vi "信号光谱4-拟合.vi"() -> ()   [LabVIEW 2015]
uses:
  <vilib>/Utility/file.llb/Write Delimited Spreadsheet (DBL).vi
  <vilib>/Analysis/NI_AALBase.lvlib
panel:
  out "范围内？":bool[](array[boolean])
  out "w":dbl
  out "xc":dbl
  out "拟合参数":dbl[](array[numeric])
  out "best fit":dbl[](graph) caption="最佳拟合"
  out "最终存储路径":path
  in  "停止程序":bool
  in  "上升下降沿/s":dbl format="%.2p"
  in  "延时/s":dbl format="%.2p"
  in  "占空比/%":dbl=3.0 format="%.2p"
  in  "高电平/V":dbl=4.0 format="%.2p"
  in  "频率/Hz":dbl=100.0 format="%.3p"
  in  "低电平/V":dbl min=0.0 max=5.0 format="%.2p"
  out "configure error out":errorcluster
  in  "设置参数":bool
  out "output control error  4":errorcluster
  in  "低电平持续输出":bool
  in  "Output 1":bool
  out "output control error  5":errorcluster
  in  "脉冲作用时间/s":dbl=1.0
  in  "测量高电平/V":dbl=4.0
  out "output control error  2":errorcluster
  in  "测量次数":i32=1
  in  "开始测量":bool
  in  "上升下降沿":i32(ring)=1 items=["上升沿", "下降沿"]
  in  "channel输出口":i32(ring) items=["Channel 1", "Channel 2"]
  in  "输出信号波形":u16(ring) items=["Pulse"]
  out "output control error  3":errorcluster
  out "Output":bool
  in  "VISA 信号发生器":refnum<visa-resource-name>="USB0::0x1AB1::0x0641::DG4E192200870::INSTR"
  out "Spectrum":cluster{"Y":dbl[], "Y":dbl[]}[](graph)
  in  "计数器":dbl=720.0
  out "波长范围":dbl[](array[numeric])
  in  "选项卡控件":enum32{"IHR 550", "CCD"}(tab)
  in  "Move To\nTarget Positions":bool
  out "Current UniqueID":string="Mono4"
  in  "Mono ID":string(combo)="Mono1"
  in  "Connect":bool
  out "Initialized JY":bool=TRUE
  in  "Force\nInitialization":bool
  in  "Target Grating":string(combo)="2"
  out "Current Description":string="1" caption="Description"
  out "Grating Index":i32=1
  out "Current Grating":dbl=1200.0
  out "Units":string="nm"
  out "Current WL":dbl=897.9988
  out "Exit Mirror\nPosition":i32(ring)=2 items=["EntranceMirror", "ExitMirror", "Front", "Side"]
  out "Entrance Mirror\nPosition":i32(ring)=2 items=["EntranceMirror", "ExitMirror", "Front", "Side"]
  out "Units 2":string="mm"
  out "Front Entrance":dbl
  in  "Target WL":dbl=2670.0
  in  "Exit Mirror":u16(ring)=3 caption="Target Position Exit Mirror" items=["Front"=2, "Side"=3]
  in  "Entrance Mirror":u16(ring)=2 caption="Target Position\nEntrance Mirror" items=["Front"=2, "Side"=3]
  in  "Target\nFront Entrance":dbl=1.0
  in  "Commande tab":T1(tab)
  in  "Area Number to Display":i32
  in  "Reformat":bool
  in  "GAIN":u16(ring)=2 caption="Device Name" items=["High Light", "Best Dynamic Range", "High Sensitivity"]
  in  "ADC":u16(ring) caption="Device Name" items=["20 kHz       ", " 1 MHz       ", " 1 MHz Ultra "]
  in  "Number of Areas :":u16=1 min=1 step=1
  in  "Integration time (ms) :":i16=5000
  out "Uniques ID":u16(ring) items=["CCD1", "CCD2"]
  in  "Device Name":u16(ring) items=["Synapse CCD (Lateral)", "Synapse_IGA (Axial)"]
  in  "Signal type :":enum16{"TTL Rising Edge", "TTL Falling Edge"}(ring)=enum."TTL Falling Edge"
  in  "Trigger Type :":u16(ring) items=["On Start"=1, "Per Acquisition"=2]
  in  "trigSigTypeString":string
  in  "trigEventString":string
  in  "Enable InputTriggers :":bool
  in  "Number of Cleans":i32=1
  in  "MultiAcqShutterMode":i32(ring)=3 items=["Open For All Spectra"=1, "Open for Each Spectrum"=3]
  in  "Accumulations:":u16=10 min=1 step=1
  in  "Multi Accumulation mode:":bool
  out "Y Pixels:":i32=256
  out "DataSize":i32=1024
  out "X Pixels:":i32=1024
  out "Firmware\nVersion":string="V1.20 CCD_4000"
  out "initialized ?":bool=TRUE
  in  "Continuous":bool
  in  "CCD Busy":bool
  out "indicator":string="Ready !"
  in  "initialize":bool
  in  "ShutterOpen":bool=TRUE caption="Shutter enable"
  in  "Acquire":bool
  in  "Temperature":bool
  in  "Setup":bool
  in  "起始波长":dbl=2406.79
  in  "终止波长":dbl=2919.91
  out "Acq Time(ms)":u32=3401
  in  "Save Backlight":bool
  in  "cut backlight":bool
  out "backlight":bool=TRUE
  in  "Close":bool=TRUE
  out "JYCCDLib.IJYCCDReqd":refnum<k7>
  out "areas :":i32[][](array[numeric])=[[1], [1], [1], [1024], [256], [1], [256]]
  in  "Constante de condition\n(Voir l'aide contextuelle)":bool
  out "temp graph":dbl(graph)=-134.538067
  out "ADC Number":i32[](array[numeric])=[0, 1, 2, 3, 4]
  out "Gain Number":i32[](array[numeric])=[10, 11, 12, 13, 8, 2]
  out "trigAddress":i32
  out "Data":i32[][](graph)
  out "error out":errorcluster
  out "Gratings":dbl[](array[numeric])=[1200.0, 300.0]
  out "Backlight":i32[][](graph)
  out "data 2":i32[][](graph)
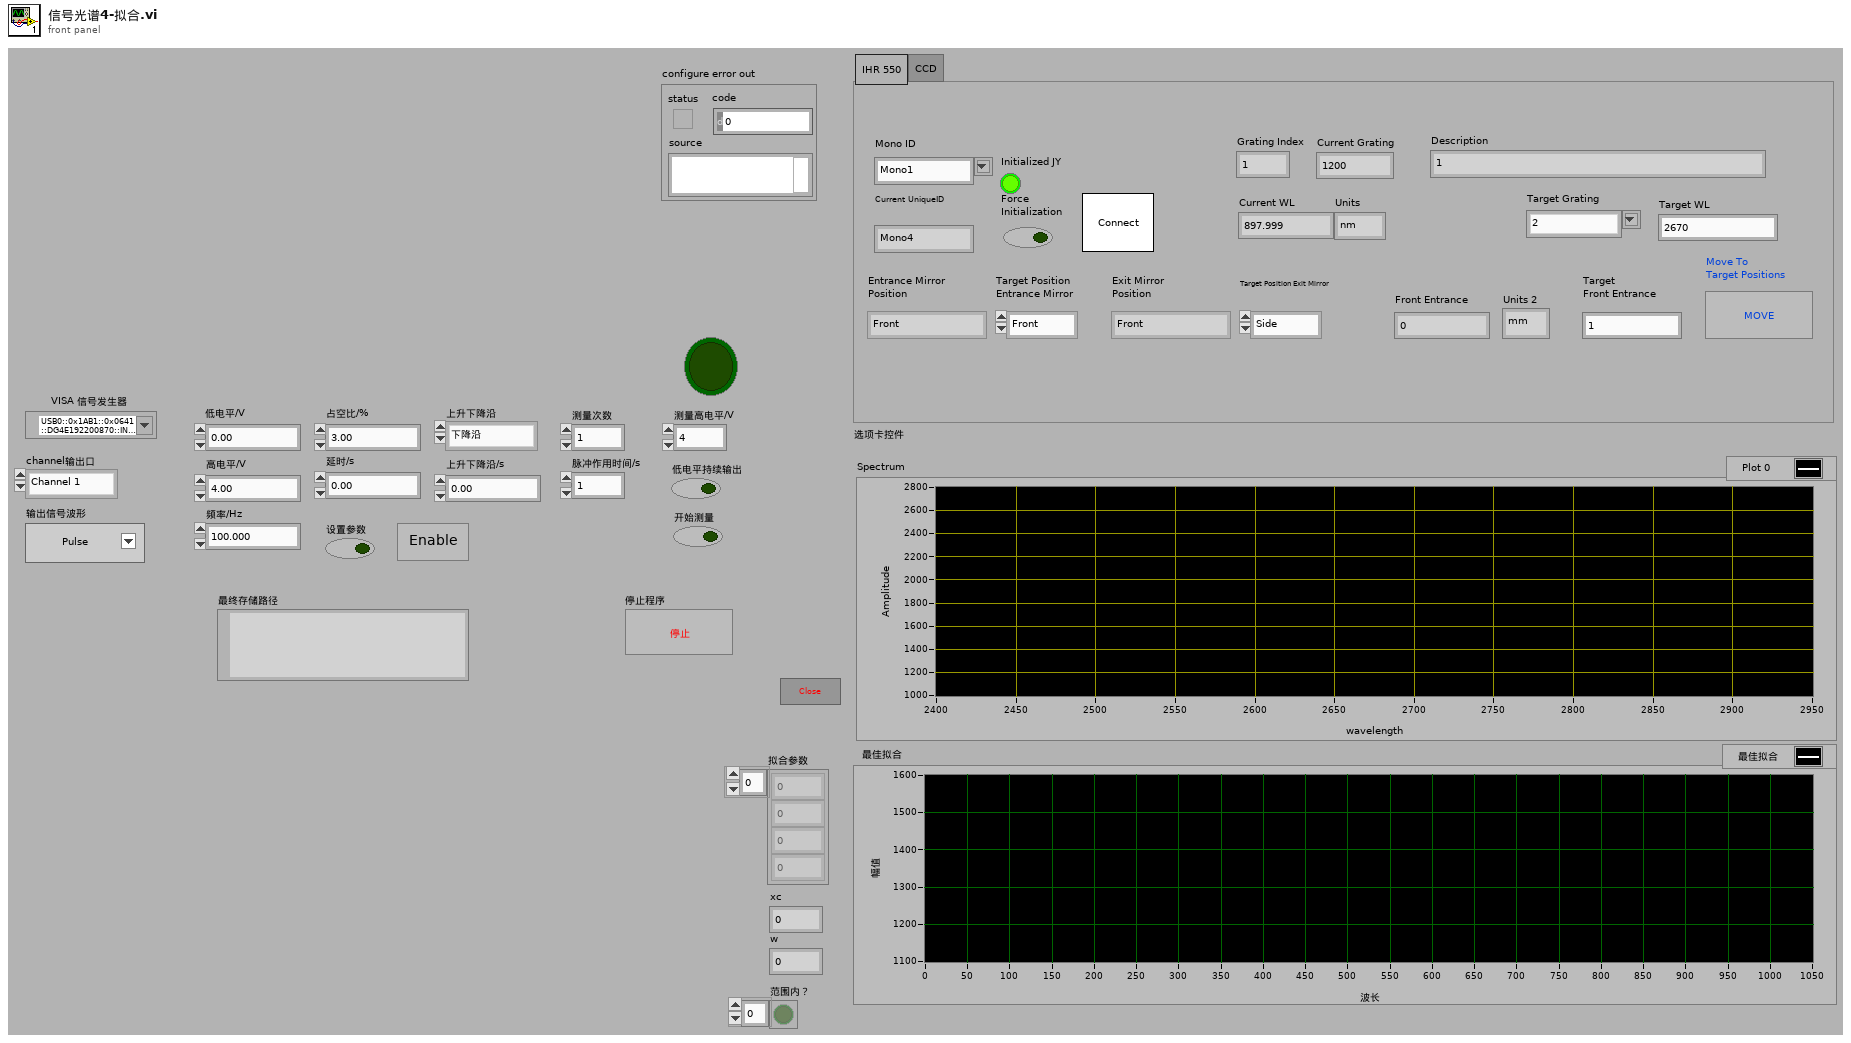
[diagram p1: front panel]
types:
  T1 = enum32{"Settings", "Trigger In", "Multi-Accu.", "Infos"}
  T2 = enum8{"Enabled", "Disabled", "Disabled and Grayed Out"}
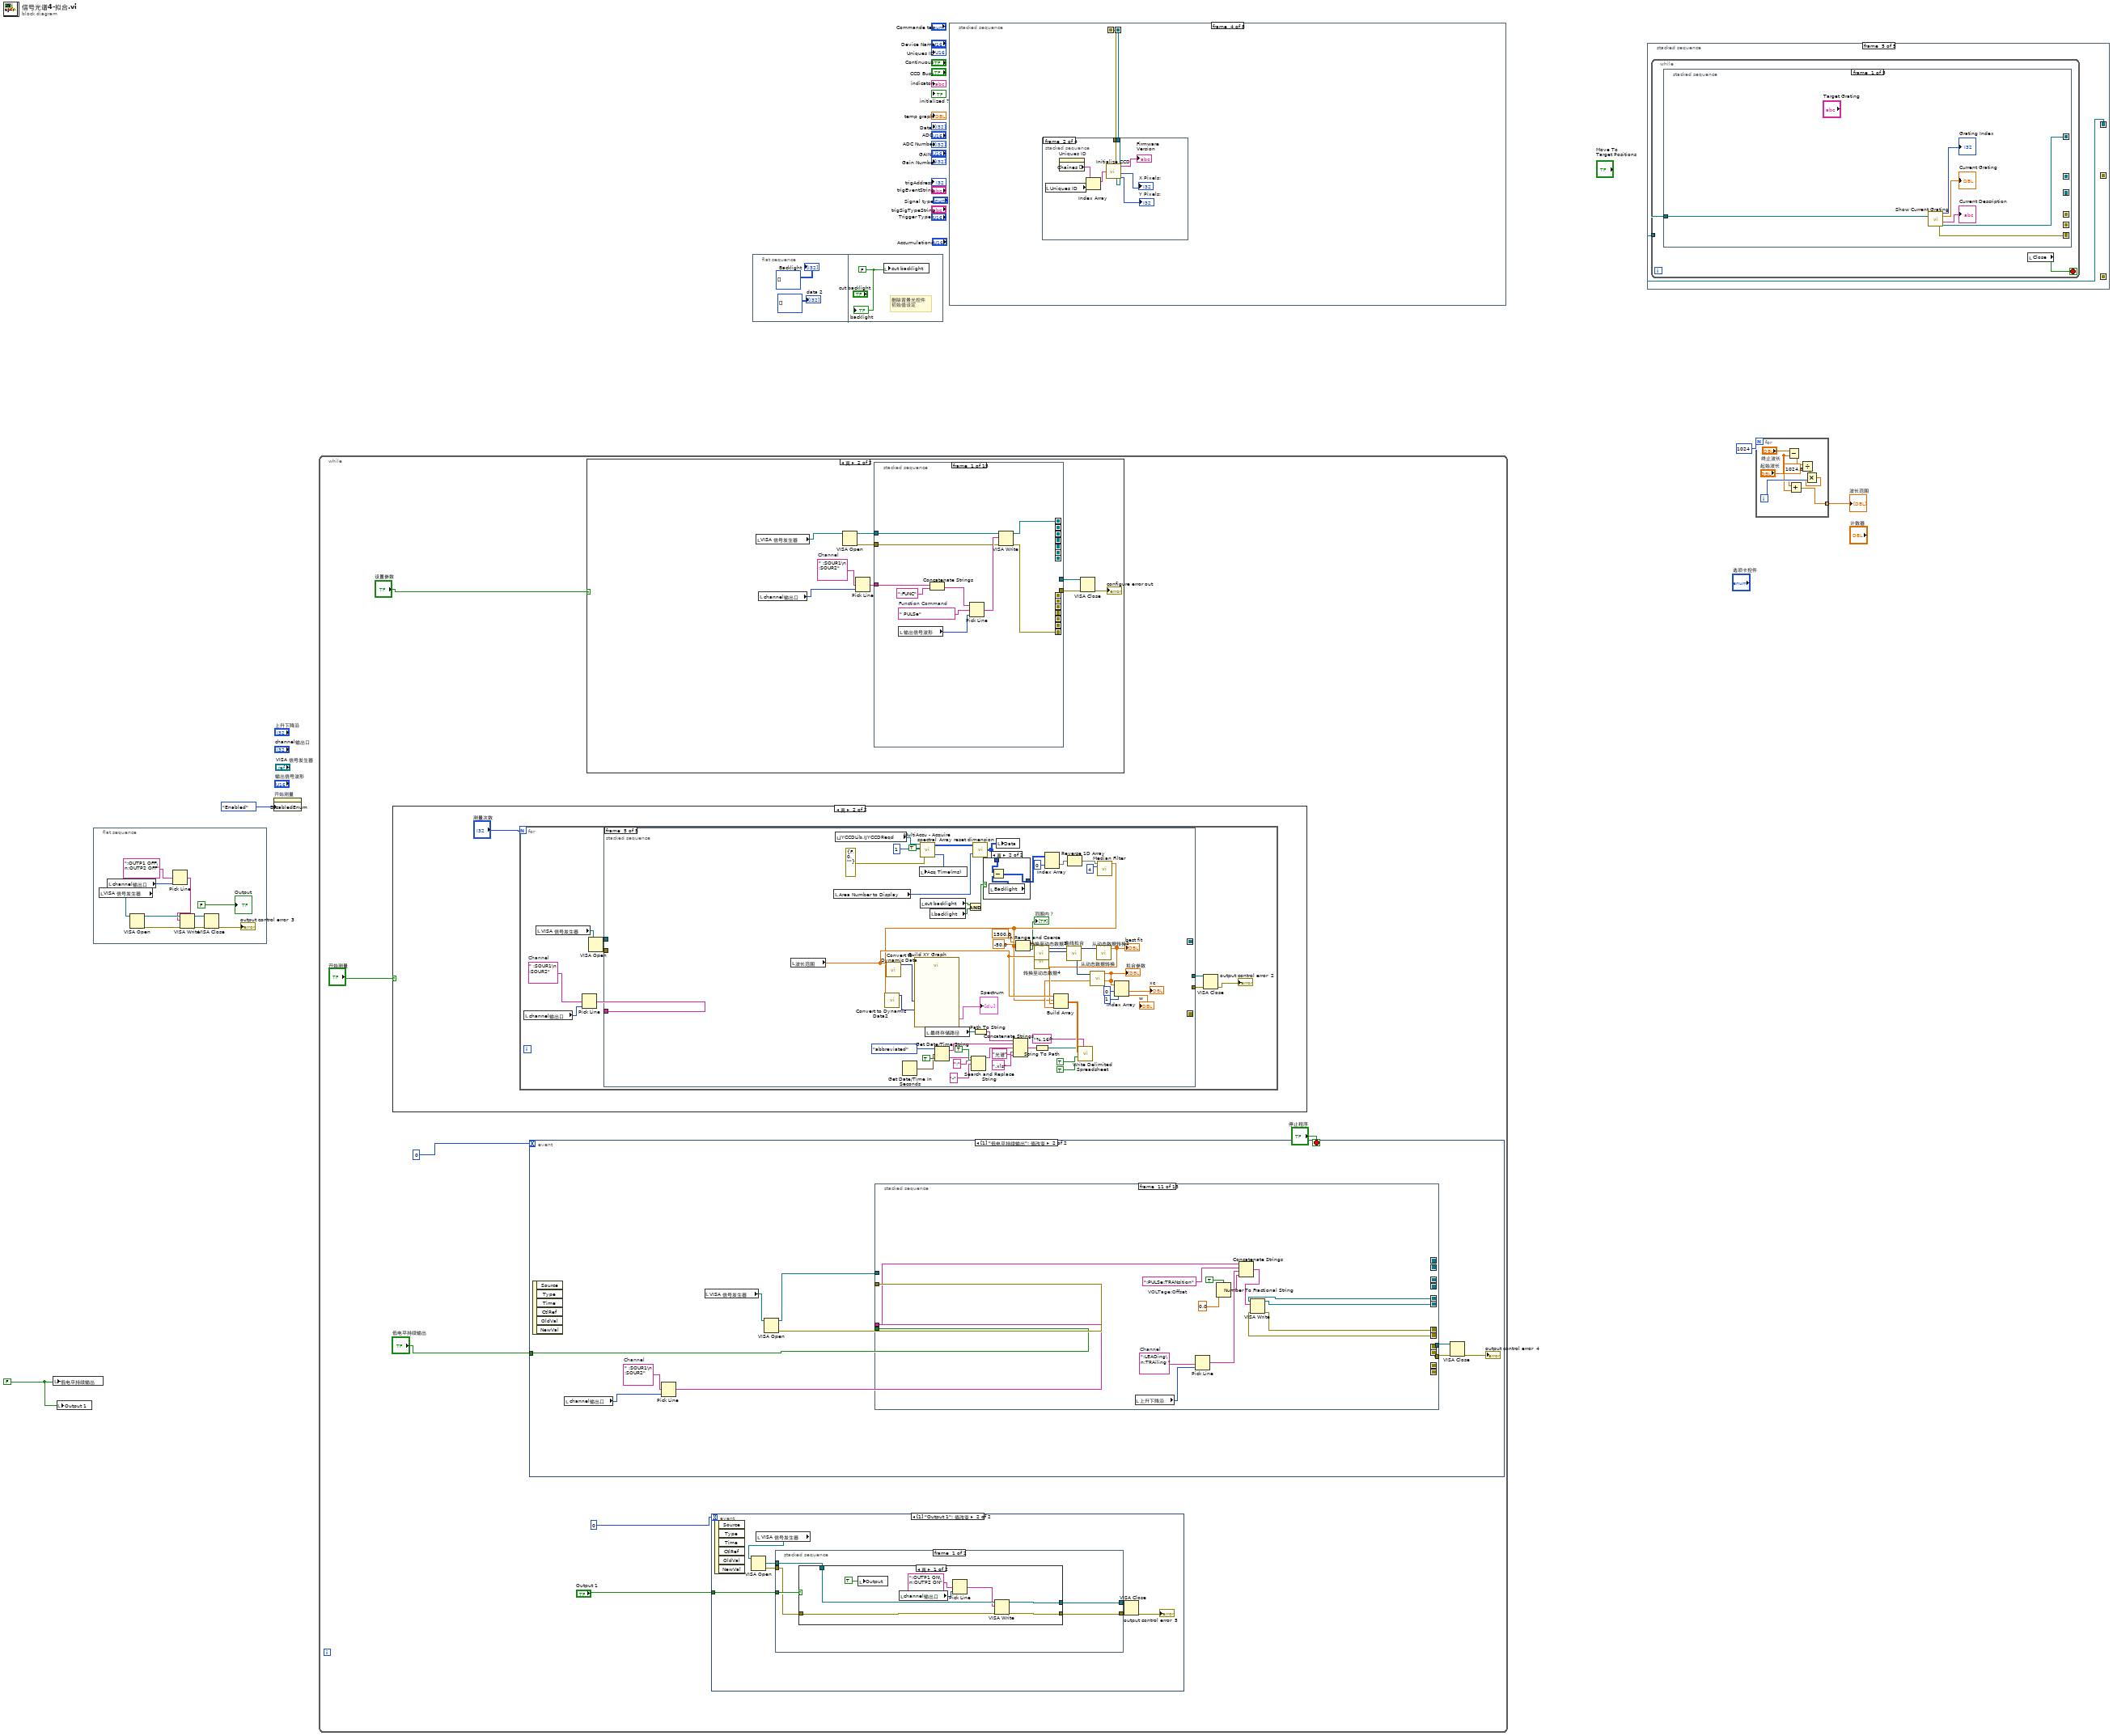
[diagram p0: block diagram]
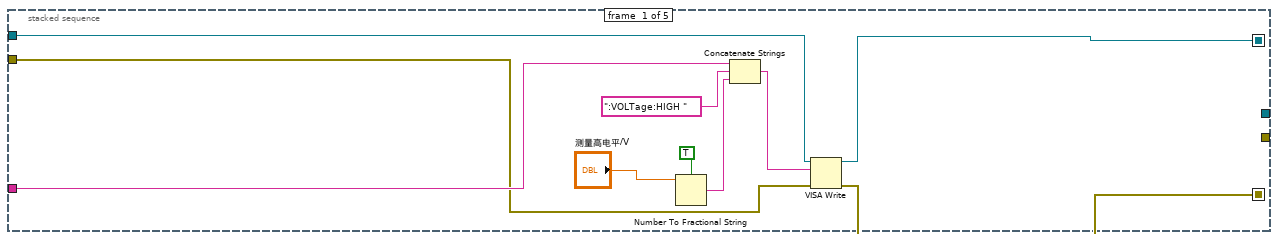
[diagram p3: hidden frame]
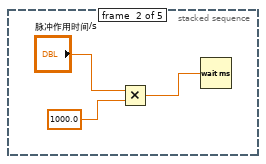
[diagram p4: hidden frame]
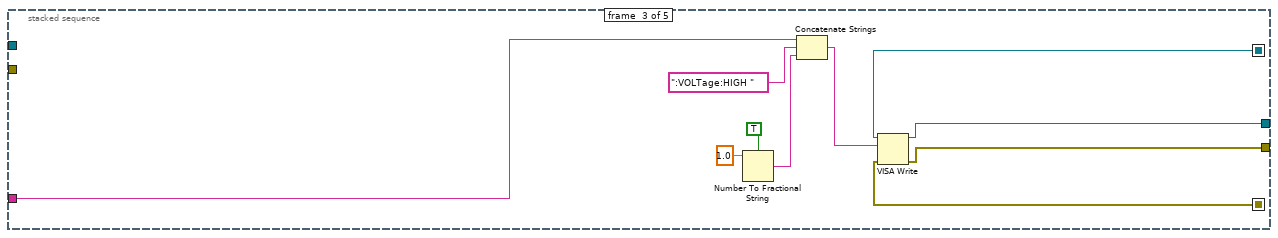
[diagram p5: hidden frame]
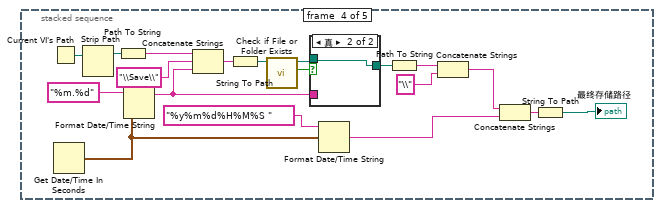
[diagram p6: hidden frame]
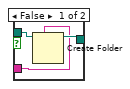
[diagram p7: hidden frame]
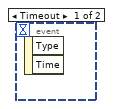
[diagram p9: hidden frame]
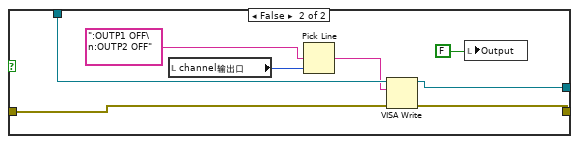
[diagram p10: hidden frame]
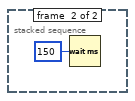
[diagram p11: hidden frame]
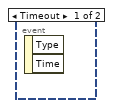
[diagram p12: hidden frame]
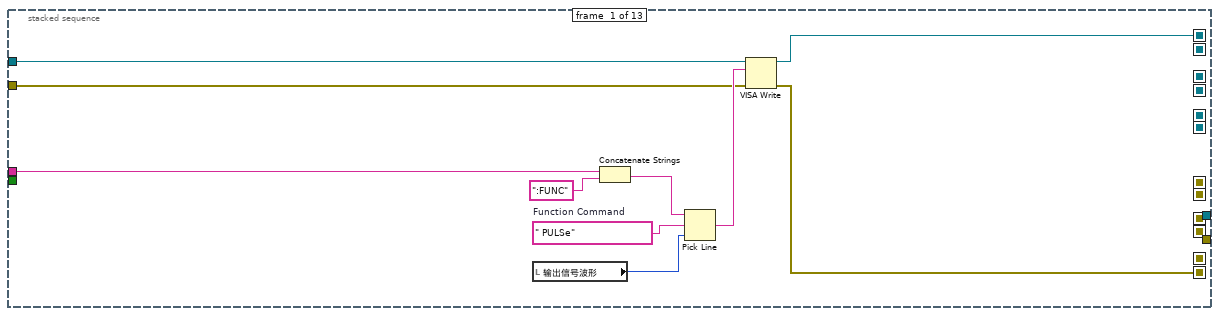
[diagram p13: hidden frame]
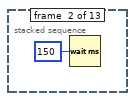
[diagram p14: hidden frame]
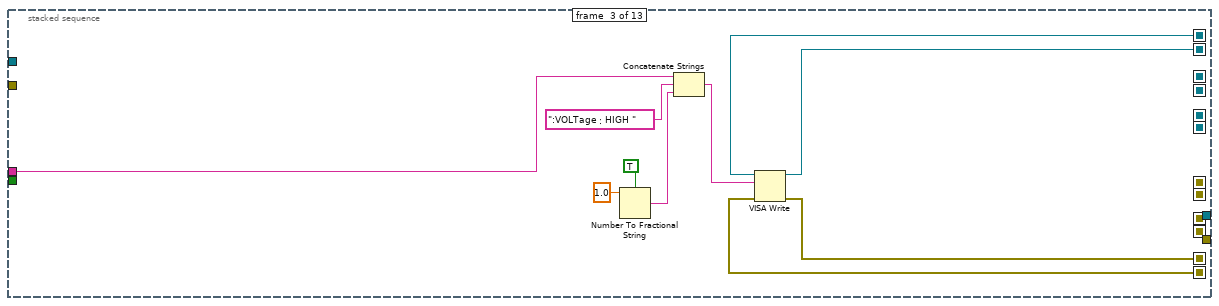
[diagram p15: hidden frame]
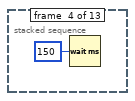
[diagram p16: hidden frame]
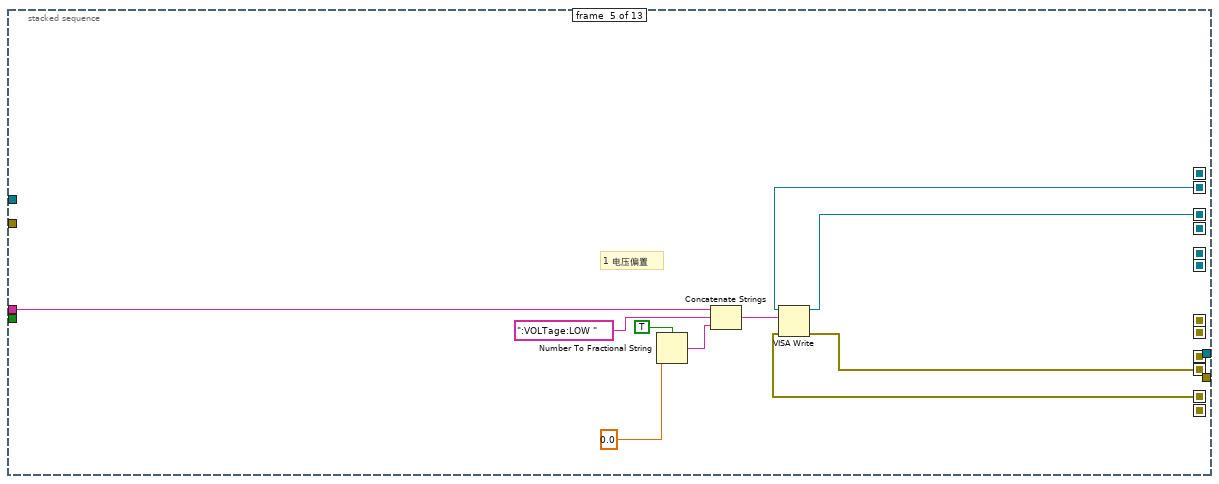
[diagram p17: hidden frame]
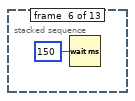
[diagram p18: hidden frame]
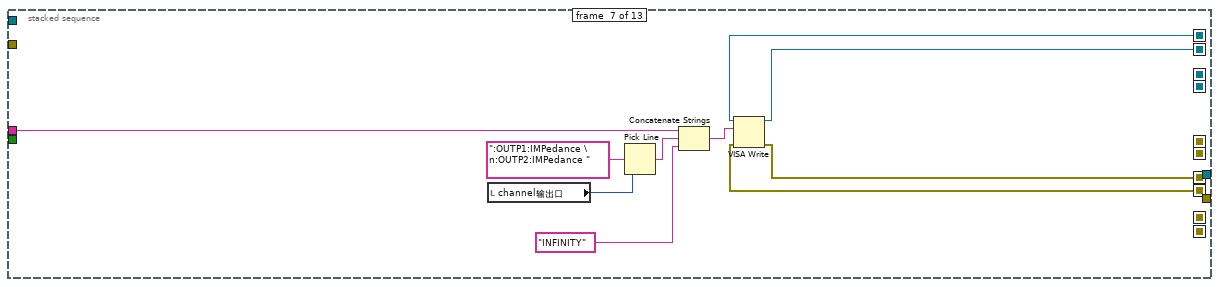
[diagram p19: hidden frame]
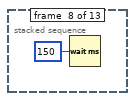
[diagram p20: hidden frame]
diagram:
  w1 = FALSE
  n1 = local write "低电平持续输出"(w1) -> ()
  n2 = local write "Output 1"(w1) -> ()
  n3 = flat-sequence {
    frame #0 {
      n4 = local read "VISA 信号发生器"() -> (w8:refnum<visa-resource-name>)
      n5 = local read "channel输出口"() -> (w6:i32)
      n6 = VISA Open(VISA resource name=w8) -> (VISA resource name=w14:refnum<visa-resource-name>, error out=w13:errorcluster)  [unwired: 4 in]
      n7 = Pick Line(multi-line string=":OUTP1 OFF\n:OUTP2 OFF" ("write buffer"), line index=w6) -> (output string=w5:string)  [unwired: 1 in]
      n8 = VISA Write(VISA resource name=w14, write buffer=w5, error in (no error)=w13) -> (VISA resource name out=w11:refnum<visa-resource-name>, error out=w10:errorcluster)  [unwired: 1 out]
      n9 = VISA Close(VISA resource name=w11, error in (no error)=w10) -> (error out=→"output control error  3":errorcluster)
      "Output" <- FALSE ("布尔")
    }
  }
  n10 = property on="开始测量" class="Bool"("DisabledEnum"=T2."Enabled" ("禁用")) -> ()  [unwired: 2 in, 2 out]
  n11 = while {
    stop <- "停止程序" stop-if-true
    n12 = case shown="真" "开始测量" {
      frame False {
      }
      frame True {
        n13 = for {
          N: "测量次数" -> [_]
          w24 = " :SOUR1\n :SOUR2"  # Channel
          n14 = local read "channel输出口"() -> (w25:i32)
          n15 = local read "VISA 信号发生器"() -> (w31:refnum<visa-resource-name>)
          n16 = Pick Line(multi-line string=w24, line index=w25) -> (output string=w23:string)  [unwired: 1 in]
          n17 = VISA Open(VISA resource name=w31) -> (VISA resource name=w30:refnum<visa-resource-name>, error out=w29:errorcluster)  [unwired: 4 in]
          n18 = stacked-sequence {
            seq-local: [w34 _ _ _ _] -> [_ _ w47 _ _]
            seq-local: [w33 _ _ _ _] -> [_ _ w46 _ _]
            tunnel: w30 -> [w36 _ _ _ _]
            tunnel: w29 -> [w35 _ _ _ _]
            tunnel: [_ _ w49 _ _] -> w28
            tunnel: [_ _ w48 _ _] -> w27
            tunnel: w23 -> [w37 _ w45 _ _]
            frame #0 {
              n19 = Number To Fractional String(use system decimal point (T)=TRUE ("使用系统小数点(T)"), number="测量高电平/V") -> (F-format string=w39:string)  [unwired: 2 in]
              n20 = Concatenate Strings ("连接字符串")(w37, ":VOLTage:HIGH ", w39) -> (w38:string)
              n21 = VISA Write(VISA resource name=w36, write buffer=w38, error in (no error)=w35) -> (VISA resource name out=w34:refnum<visa-resource-name>, error out=w33:errorcluster)  [unwired: 1 out]
            }
            frame #1 {
              n22 = Multiply(x="脉冲作用时间/s", y=1000.0) -> (x*y=w42:dbl)
              n23 = Wait (ms)(milliseconds to wait=w42) -> ()  [unwired: 1 out]
            }
            frame #2 {
              n24 = Number To Fractional String(use system decimal point (T)=TRUE ("使用系统小数点(T)"), number=1.0 ("数字")) -> (F-format string=w52:string)  [unwired: 2 in]
              n25 = Concatenate Strings ("连接字符串")(w45, ":VOLTage:HIGH ", w52) -> (w51:string)
              n26 = VISA Write(VISA resource name=w47, write buffer=w51, error in (no error)=w46) -> (VISA resource name out=w49:refnum<visa-resource-name>, error out=w48:errorcluster)  [unwired: 1 out]
            }
            frame #3 {
              n27 = Current VI's Path() -> (path=w60:path)
              n28 = Get Date/Time In Seconds() -> (seconds since 1Jan1904=w62:timestamp)
              n29 = Strip Path(path=w60) -> (stripped path=w61:path)  [unwired: 1 out]
              n30 = Path To String(path=w61) -> (string=w63:string)
              n31 = Format Date/Time String(time format string (%c)="%m.%d" ("时间格式字符串(%c)"), seconds (now)=w62) -> (date/time string=w69:string)  [unwired: 1 in]
              n32 = Concatenate Strings(w63, "\\Save\\" ("字符串"), w69) -> (w64:string)
              n33 = String To Path(string=w64) -> (path=w65:path)
              n34 = call <vilib>:"Check if File or Folder Exists.vi"("path"=w65) -> ("file or folder exists?"=w66:bool, "dup path"=w68:path)  [unwired: 8 in, 1 out]
              n35 = case shown="真" w66 {
                tunnel: [w76 w77] -> w67
                tunnel: w68 -> [w75 w77]
                tunnel: w69 -> [w74 _]
                frame False {
                  n36 = Create Folder(prompt (Create Folder)=w74, path (use dialog)=w75) -> (created path=w76:path)  [unwired: 1 in, 2 out]
                }
                frame True {
                }
              }
              n37 = Format Date/Time String(time format string (%c)="%y%m%d%H%M%S " ("时间格式字符串(%c)"), seconds (now)=w62) -> (date/time string=w72:string)  [unwired: 1 in]
              n38 = Path To String(path=w67) -> (string=w70:string)
              n39 = Concatenate Strings(w70, "\\" ("字符串")) -> (w71:string)
              n40 = Concatenate Strings(w71, w72) -> (w59:string)
              n41 = String To Path(string=w59) -> (path=→"最终存储路径":path)
            }
            frame #4 {
              n42 = local read "波长范围"() -> (w95:dbl[])
              n43 = local read "Area Number to Display"() -> (w105:i32)
              n44 = local read "JYCCDLib.IJYCCDReqd"() -> (w101:refnum<k7>)
              n45 = call "Convert to Dynamic Data"("Array"=w95) -> ("Dynamic Data Type"=w98:dynamicdata)  [unwired: 3 in]
              n46 = Get Date/Time In Seconds() -> (seconds since 1Jan1904=w114:timestamp)
              n47 = call <userlib>:"MultiAccu - Acquire spectral.vi"("error in"=errorcluster {"status"=FALSE, "code"=0, "source"=""}, "Accumulations:"=u16 1, "ShutterOpen"=TRUE, "JYCCDLib.IJYCCDReqd"=w101) -> ("Acq Time(ms)"=w107:u32, "Array Out"=w106:i32[][][])  [unwired: 1 out]
              n48 = local write "Acq Time(ms)"(w107) -> ()
              n49 = local read "cut backlight"() -> (w85:bool)
              n50 = local read "最终存储路径"() -> (w128:path)
              n51 = local read "backlight"() -> (w83:bool)
              n52 = Get Date/Time String(date format (0)=enum16{"short", "long", "abbreviated"}."abbreviated" ("日期格式(0)"), seconds (now)=w114, want seconds? (F)=TRUE ("需要秒？(F)")) -> (date string=w122:string, time string=w117:string)
              n53 = And(x=w85, y=w83) -> (x .and. y?=w84:bool)
              n54 = Search and Replace String(replace all?=TRUE ("替换全部？(F)"), input string=w117, search string=":" ("搜索字符串"), replace string="-" ("替换字符串(\"\")")) -> (result string=w121:string)  [unwired: 4 in, 3 out]
              n55 = call <userlib>:"Array reset dimension.vi"("Area Number"=w105, "Array In"=w106) -> ("Array Out"=w87:i32[][])
              n56 = Path To String(path=w128) -> (string=w111:string)
              n57 = case shown="真" w84 {
                tunnel: [w132 w134] -> w86
                tunnel: w87 -> [w132 w133]
                frame False {
                }
                frame True {
                  n58 = local read "Backlight"() -> (w135:i32[][])
                  n59 = Subtract(x=w133, y=w135) -> (x-y=w134:i32[][])
                }
              }
              n60 = local write "Data"(w87) -> ()
              n61 = Concatenate Strings(w111, w122, w121, "光谱" ("字符串"), ".xls" ("字符串")) -> (w126:string)
              n62 = call "转换至动态数据4"("Array"=w95) -> ("Dynamic Data Type"=w94:dynamicdata)  [unwired: 3 in]
              n63 = String To Path(string=w126) -> (path=w127:path)
              n64 = Index Array(array=w86, index (row)=0 ("索引 (行)")) -> (element=w129:i32[])  [unwired: 1 in]
              n65 = Reverse 1D Array(array=w129) -> (reversed array=w130:i32[])
              n66 = call <vilib>:"Median Filter.vi"("left rank"=4, "X"=w130) -> ("Filtered X"=w82:dbl[])  [unwired: 8 in, 1 out]
              n67 = call "Convert to Dynamic Data2"("Array"=w82) -> ("Dynamic Data Type"=w97:dynamicdata)  [unwired: 3 in]
              n68 = call "Build XY Graph"("Y Input"=w97, "X Input"=w98) -> ("XY Graph"=→"Spectrum":cluster{"Y":dbl[], "Y":dbl[]}[])  [unwired: 8 in, 1 out]
              n69 = In Range and Coerce(upper limit=1500.0, x=w82, lower limit=-50.0) -> (coerced(x)=w79:dbl[], In Range?=→"范围内？":bool[])
              n70 = call "转换至动态数据3"("Array"=w79) -> ("Dynamic Data Type"=w96:dynamicdata)  [unwired: 3 in]
              n71 = call "曲线拟合"("Locations"=w94, "Signals"=w96) -> ("best fit"=w100:dynamicdata, "non-linear coefficients"=w99:dynamicdata)  [unwired: 5 in, 3 out]
              n72 = call "从动态数据转换"("Dynamic Data Type"=w99) -> ("Array"=w90:dbl[])  [unwired: 3 in]
              "拟合参数" <- w90
              n73 = call "从动态数据转换2"("Dynamic Data Type"=w100) -> ("Array"=w91:dbl[])  [unwired: 3 in]
              "best fit" <- w91
              n74 = Build Array(w95, w82, w91, w90) -> (w131:dbl[][])
              n75 = call-poly <vilib>:"Write Delimited Spreadsheet.vi"("file path (dialog if empty)"=w127, "format (%.3f)"="%.16f", "2D data"=w131, "append to file? (F)"=TRUE, "transpose? (F)"=TRUE) -> ()  [unwired: 9 in, 2 out]
              n76 = Index Array(array=w90, index #1=0 ("索引"), index #2=1 ("索引")) -> (element #1=→"xc":dbl, element #2=→"w":dbl)
            }
          }
          n77 = VISA Close(VISA resource name=w28, error in (no error)=w27) -> (error out=→"output control error  2":errorcluster)
        }
      }
    }
    n78 = event shown="[1] \"低电平持续输出\": 值改变" {
      selector: _ -> [_ _]
      dyn-events: _ -> [_ _]
      timeout: u32 0 ("Time") -> [_ _]
      tunnel: "低电平持续输出" -> [_ w165]
      event Timeout {
        n79 = event-data() -> ()  [unwired: 1 in, 2 out]
      }
      event "低电平持续输出": Value Change {
        w169 = " :SOUR1\n :SOUR2"  # Channel
        n80 = event-data() -> ()  [unwired: 1 in, 6 out]
        n81 = local read "channel输出口"() -> (w170:i32)
        n82 = Pick Line(multi-line string=w169, line index=w170) -> (output string=w168:string)  [unwired: 1 in]
        n83 = local read "VISA 信号发生器"() -> (w173:refnum<visa-resource-name>)
        n84 = VISA Open(VISA resource name=w173) -> (VISA resource name=w172:refnum<visa-resource-name>, error out=w171:errorcluster)  [unwired: 4 in]
        n85 = stacked-sequence {
          seq-local: [w179 _ _ _ _ _ _ _ _ _ _ _ _] -> [_ _ w194 _ _ _ _ _ _ _ _ _ _]
          seq-local: [w178 _ _ _ _ _ _ _ _ _ _ _ _] -> [_ _ w193 _ _ _ _ _ _ _ _ _ _]
          seq-local: [_ _ w192 _ _ _ _ _ _ _ _ _ _] -> [_ _ _ _ w197 _ _ _ _ _ _ _ _]
          seq-local: [_ _ w191 _ _ _ _ _ _ _ _ _ _] -> [_ _ _ _ w198 _ _ _ _ _ _ _ _]
          seq-local: [_ _ _ _ w206 _ _ _ _ _ _ _ _] -> [_ _ _ _ _ _ w217 _ _ _ _ _ _]
          seq-local: [_ _ _ _ w205 _ _ _ _ _ _ _ _] -> [_ _ _ _ _ _ w216 _ _ _ _ _ _]
          seq-local: [_ _ _ _ _ _ w210 _ _ _ _ _ _] -> [_ _ _ _ _ _ _ _ w220 _ _ _ _]
          seq-local: [_ _ _ _ _ _ w209 _ _ _ _ _ _] -> [_ _ _ _ _ _ _ _ w219 _ _ _ _]
          seq-local: [_ _ _ _ _ _ _ _ w223 _ _ _ _] -> [_ _ _ _ _ _ _ _ _ _ w234 _ _]
          seq-local: [_ _ _ _ _ _ _ _ w222 _ _ _ _] -> [_ _ _ _ _ _ _ _ _ _ w233 _ _]
          seq-local: [_ _ _ _ _ _ _ _ _ _ w231 _ _] -> [_ _ _ _ _ _ _ _ _ _ _ _ w248]
          seq-local: [_ _ _ _ _ _ _ _ _ _ w230 _ _] -> [_ _ _ _ _ _ _ _ _ _ _ _ w247]
          tunnel: w172 -> [w184 _ _ _ _ _ _ _ _ _ _ _ _]
          tunnel: w171 -> [w177 _ _ _ _ _ _ _ _ _ _ _ _]
          tunnel: w168 -> [w176 _ w190 _ w203 _ w214 _ w224 _ w237 _ _]
          tunnel: [_ _ _ _ _ _ _ _ _ _ _ _ w246] -> w167
          tunnel: [_ _ _ _ _ _ _ _ _ _ _ _ w244] -> w166
          tunnel: w165 -> [_ _ _ _ _ _ _ _ _ _ _ _ w245]
          frame #0 {
            w181 = " PULSe"  # Function Command
            n86 = local read "输出信号波形"() -> (w175:u16)
            n87 = Concatenate Strings(w176, ":FUNC" ("string (\"\")")) -> (w182:string)
            n88 = Pick Line(string ("")=w182, multi-line string=w181, line index=w175) -> (output string=w180:string)
            n89 = VISA Write(VISA resource name=w184, write buffer=w180, error in (no error)=w177) -> (VISA resource name out=w179:refnum<visa-resource-name>, error out=w178:errorcluster)  [unwired: 1 out]
          }
          frame #1 {
            n90 = Wait (ms)(milliseconds to wait=u32 150) -> ()  [unwired: 1 out]
          }
          frame #2 {
            n91 = Number To Fractional String(use system decimal point (T)=TRUE ("使用系统小数点(T)"), number=1.0 ("数字")) -> (F-format string=w188:string)  [unwired: 2 in]
            n92 = Concatenate Strings ("连接字符串")(w190, ":VOLTage：HIGH ", w188) -> (w187:string)
            n93 = VISA Write(VISA resource name=w194, write buffer=w187, error in (no error)=w193) -> (VISA resource name out=w192:refnum<visa-resource-name>, error out=w191:errorcluster)  [unwired: 1 out]
          }
          frame #3 {
            n94 = Wait (ms)(milliseconds to wait=u32 150) -> ()  [unwired: 1 out]
          }
          frame #4 {
            # "1 电压偏置"
            n95 = Number To Fractional String(use system decimal point (T)=TRUE ("使用系统小数点(T)"), number=0.0 ("数字")) -> (F-format string=w201:string)  [unwired: 2 in]
            n96 = Concatenate Strings(w203, ":VOLTage:LOW ", w201) -> (w202:string)
            n97 = VISA Write(VISA resource name=w197, write buffer=w202, error in (no error)=w198) -> (VISA resource name out=w206:refnum<visa-resource-name>, error out=w205:errorcluster)  [unwired: 1 out]
          }
          frame #5 {
            n98 = Wait (ms)(milliseconds to wait=u32 150) -> ()  [unwired: 1 out]
          }
          frame #6 {
            n99 = local read "channel输出口"() -> (w212:i32)
            n100 = Pick Line(multi-line string=":OUTP1:IMPedance \n:OUTP2:IMPedance " ("write buffer"), line index=w212) -> (output string=w211:string)  [unwired: 1 in]
            n101 = Concatenate Strings ("连接字符串")(w214, w211, "INFINITY") -> (w215:string)
            n102 = VISA Write(VISA resource name=w217, write buffer=w215, error in (no error)=w216) -> (VISA resource name out=w210:refnum<visa-resource-name>, error out=w209:errorcluster)  [unwired: 1 out]
          }
          frame #7 {
            n103 = Wait (ms)(milliseconds to wait=u32 150) -> ()  [unwired: 1 out]
          }
          frame #8 {
            n104 = Number To Fractional String(use system decimal point (T)=TRUE ("使用系统小数点(T)"), number=0.0 ("数字")) -> (F-format string=w227:string)  [unwired: 2 in]
            n105 = Concatenate Strings(w224, ":PULSe:DELay ", w227) -> (w225:string)
            n106 = VISA Write(VISA resource name=w220, write buffer=w225, error in (no error)=w219) -> (VISA resource name out=w223:refnum<visa-resource-name>, error out=w222:errorcluster)  [unwired: 1 out]
          }
          frame #9 {
            n107 = Wait (ms)(milliseconds to wait=u32 150) -> ()  [unwired: 1 out]
          }
          frame #10 {
            w238 = ":LEADing\n:TRAiling "  # Channel
            w242 = ":PULSe:TRANsition"  # VOLTage:Offset
            n108 = local read "上升下降沿"() -> (w239:i32)
            n109 = Pick Line(multi-line string=w238, line index=w239) -> (output string=w235:string)  [unwired: 1 in]
            n110 = Number To Fractional String(use system decimal point (T)=TRUE ("使用系统小数点(T)"), number=0.0 ("数字")) -> (F-format string=w236:string)  [unwired: 2 in]
            n111 = Concatenate Strings(w237, w242, w235, w236) -> (w240:string)
            n112 = VISA Write(VISA resource name=w234, write buffer=w240, error in (no error)=w233) -> (VISA resource name out=w231:refnum<visa-resource-name>, error out=w230:errorcluster)  [unwired: 1 out]
          }
          frame #11 {
            n113 = Wait (ms)(milliseconds to wait=u32 150) -> ()  [unwired: 1 out]
          }
          frame #12 {
            n114 = case shown="假" w245 {
              tunnel: w248 -> [w256 w257]
              tunnel: [w255 w264] -> w244
              tunnel: w247 -> [w254 w262]
              tunnel: [w253 w263] -> w246
              frame True {
                n115 = local write "Output"(TRUE ("布尔")) -> ()
                n116 = local read "channel输出口"() -> (w250:i32)
                n117 = Pick Line(multi-line string=":OUTP1 ON\n:OUTP2 ON" ("write buffer"), line index=w250) -> (output string=w249:string)  [unwired: 1 in]
                n118 = VISA Write(VISA resource name=w256, write buffer=w249, error in (no error)=w254) -> (VISA resource name out=w253:refnum<visa-resource-name>, error out=w255:errorcluster)  [unwired: 1 out]
              }
              frame False {
                n119 = local read "channel输出口"() -> (w259:i32)
                n120 = Pick Line(multi-line string=":OUTP1 OFF\n:OUTP2 OFF" ("write buffer"), line index=w259) -> (output string=w258:string)  [unwired: 1 in]
                n121 = VISA Write(VISA resource name=w257, write buffer=w258, error in (no error)=w262) -> (VISA resource name out=w263:refnum<visa-resource-name>, error out=w264:errorcluster)  [unwired: 1 out]
                n122 = local write "Output"(FALSE ("布尔")) -> ()
              }
            }
          }
        }
        n123 = VISA Close(VISA resource name=w167, error in (no error)=w166) -> (error out=→"output control error  4":errorcluster)
      }
    }
    n124 = case shown="真" "设置参数" {
      frame False {
      }
      frame True {
        w270 = " :SOUR1\n :SOUR2"  # Channel
        n125 = local read "VISA 信号发生器"() -> (w266:refnum<visa-resource-name>)
        n126 = local read "channel输出口"() -> (w265:i32)
        n127 = VISA Open(VISA resource name=w266) -> (VISA resource name=w272:refnum<visa-resource-name>, error out=w273:errorcluster)  [unwired: 4 in]
        n128 = Pick Line(multi-line string=w270, line index=w265) -> (output string=w269:string)  [unwired: 1 in]
        n129 = stacked-sequence {
          seq-local: [w278 _ _ _ _ _ _ _ _ _ _ _ _ _ _] -> [_ _ w293 _ _ _ _ _ _ _ _ _ _ _ _]
          seq-local: [w277 _ _ _ _ _ _ _ _ _ _ _ _ _ _] -> [_ _ w292 _ _ _ _ _ _ _ w331 _ _ _ _]
          seq-local: [_ _ w291 _ _ _ _ _ _ _ _ _ _ _ _] -> [_ _ _ _ w302 _ _ _ _ _ _ _ _ _ _]
          seq-local: [_ _ w290 _ _ _ _ _ _ _ _ _ _ _ _] -> [_ _ _ _ w301 _ _ _ _ _ _ _ _ _ _]
          seq-local: [_ _ _ _ w300 _ _ _ _ _ _ _ _ _ _] -> [_ _ _ _ _ _ w308 _ _ _ _ _ _ _ _]
          seq-local: [_ _ _ _ w297 _ _ _ _ _ _ _ _ _ _] -> [_ _ _ _ _ _ w307 _ _ _ _ _ _ _ _]
          seq-local: [_ _ _ _ _ _ w315 _ _ _ _ _ _ _ _] -> [_ _ _ _ _ _ _ _ w326 _ _ _ _ _ _]
          seq-local: [_ _ _ _ _ _ w314 _ _ _ _ _ _ _ _] -> [_ _ _ _ _ _ _ _ w325 _ _ _ _ _ _]
          seq-local: [_ _ _ _ _ _ _ _ w319 _ _ _ _ _ _] -> [_ _ _ _ _ _ _ _ _ _ w332 _ _ _ _]
          seq-local: [_ _ _ _ _ _ _ _ w318 _ _ _ _ _ _] -> [_ _ _ _ _ _ _ _ _ _ _ _ _ _ _]
          seq-local: [_ _ _ _ _ _ _ _ _ _ w328 _ _ _ _] -> [_ _ _ _ _ _ _ _ _ _ _ _ w342 _ _]
          seq-local: [_ _ _ _ _ _ _ _ _ _ w329 _ _ _ _] -> [_ _ _ _ _ _ _ _ _ _ _ _ w341 _ _]
          seq-local: [_ _ _ _ _ _ _ _ _ _ _ _ w340 _ _] -> [_ _ _ _ _ _ _ _ _ _ _ _ _ _ w353]
          seq-local: [_ _ _ _ _ _ _ _ _ _ _ _ w339 _ _] -> [_ _ _ _ _ _ _ _ _ _ _ _ _ _ w352]
          tunnel: w272 -> [w283 _ _ _ _ _ _ _ _ _ _ _ _ _ _]
          tunnel: w273 -> [w276 _ _ _ _ _ _ _ _ _ _ _ _ _ _]
          tunnel: w269 -> [w275 _ w289 _ w296 _ w312 _ w323 _ w333 _ w343 _ w356]
          tunnel: [_ _ _ _ _ _ _ _ _ _ _ _ _ _ w351] -> w268
          tunnel: [_ _ _ _ _ _ _ _ _ _ _ _ _ _ w350] -> w267
          frame #0 {
            w280 = " PULSe"  # Function Command
            n130 = local read "输出信号波形"() -> (w274:u16)
            n131 = Concatenate Strings(w275, ":FUNC" ("string (\"\")")) -> (w281:string)
            n132 = Pick Line(string ("")=w281, multi-line string=w280, line index=w274) -> (output string=w279:string)
            n133 = VISA Write(VISA resource name=w283, write buffer=w279, error in (no error)=w276) -> (VISA resource name out=w278:refnum<visa-resource-name>, error out=w277:errorcluster)  [unwired: 1 out]
          }
          frame #1 {
            n134 = Wait (ms)(milliseconds to wait=u32 150) -> ()  [unwired: 1 out]
          }
          frame #2 {
            n135 = Number To Fractional String(use system decimal point (T)=TRUE ("使用系统小数点(T)"), number="低电平/V") -> (F-format string=w287:string)  [unwired: 2 in]
            n136 = Concatenate Strings ("连接字符串")(w289, ":VOLTage:LOW ", w287) -> (w286:string)
            n137 = VISA Write(VISA resource name=w293, write buffer=w286, error in (no error)=w292) -> (VISA resource name out=w291:refnum<visa-resource-name>, error out=w290:errorcluster)  [unwired: 1 out]
          }
          frame #3 {
            n138 = Wait (ms)(milliseconds to wait=u32 150) -> ()  [unwired: 1 out]
          }
          frame #4 {
            # "1 频率"
            n139 = Concatenate Strings(w296, ":FREQ ") -> (w303:string)
            n140 = Format Into String ("格式化写入字符串")(initial string=w303, "频率/Hz") -> (resulting string=w304:string)  [unwired: 2 in, 1 out]
            n141 = VISA Write(VISA resource name=w302, write buffer=w304, error in (no error)=w301) -> (VISA resource name out=w300:refnum<visa-resource-name>, error out=w297:errorcluster)  [unwired: 1 out]
          }
          frame #5 {
            n142 = Wait (ms)(milliseconds to wait=u32 150) -> ()  [unwired: 1 out]
          }
          frame #6 {
            n143 = Number To Fractional String(use system decimal point (T)=TRUE ("使用系统小数点(T)"), number="高电平/V") -> (F-format string=w309:string)  [unwired: 2 in]
            n144 = Concatenate Strings(w312, ":VOLTage:HIGH ", w309) -> (w311:string)
            n145 = VISA Write(VISA resource name=w308, write buffer=w311, error in (no error)=w307) -> (VISA resource name out=w315:refnum<visa-resource-name>, error out=w314:errorcluster)  [unwired: 1 out]
          }
          frame #7 {
            n146 = Wait (ms)(milliseconds to wait=u32 150) -> ()  [unwired: 1 out]
          }
          frame #8 {
            n147 = local read "channel输出口"() -> (w321:i32)
            n148 = Pick Line(multi-line string=":OUTP1:IMPedance \n:OUTP2:IMPedance " ("write buffer"), line index=w321) -> (output string=w320:string)  [unwired: 1 in]
            n149 = Concatenate Strings ("连接字符串")(w323, w320, "INFINITY") -> (w324:string)
            n150 = VISA Write(VISA resource name=w326, write buffer=w324, error in (no error)=w325) -> (VISA resource name out=w319:refnum<visa-resource-name>, error out=w318:errorcluster)  [unwired: 1 out]
          }
          frame #9 {
            n151 = Wait (ms)(milliseconds to wait=u32 150) -> ()  [unwired: 1 out]
          }
          frame #10 {
            n152 = Number To Fractional String(use system decimal point (T)=TRUE ("使用系统小数点(T)"), number="占空比/%") -> (F-format string=w335:string)  [unwired: 2 in]
            n153 = Concatenate Strings(w333, ":PULSe:DCYCle ", w335) -> (w330:string)
            n154 = VISA Write(VISA resource name=w332, write buffer=w330, error in (no error)=w331) -> (VISA resource name out=w328:refnum<visa-resource-name>, error out=w329:errorcluster)  [unwired: 1 out]
          }
          frame #11 {
            n155 = Wait (ms)(milliseconds to wait=u32 150) -> ()  [unwired: 1 out]
          }
          frame #12 {
            n156 = Number To Fractional String(use system decimal point (T)=TRUE ("使用系统小数点(T)"), number="延时/s") -> (F-format string=w346:string)  [unwired: 2 in]
            n157 = Concatenate Strings(w343, ":PULSe:DELay ", w346) -> (w344:string)
            n158 = VISA Write(VISA resource name=w342, write buffer=w344, error in (no error)=w341) -> (VISA resource name out=w340:refnum<visa-resource-name>, error out=w339:errorcluster)  [unwired: 1 out]
          }
          frame #13 {
            n159 = Wait (ms)(milliseconds to wait=u32 150) -> ()  [unwired: 1 out]
          }
          frame #14 {
            w357 = ":LEADing\n:TRAiling "  # Channel
            w362 = ":PULSe:TRANsition"  # VOLTage:Offset
            n160 = local read "上升下降沿"() -> (w358:i32)
            n161 = Pick Line(multi-line string=w357, line index=w358) -> (output string=w354:string)  [unwired: 1 in]
            n162 = Number To Fractional String(use system decimal point (T)=TRUE ("使用系统小数点(T)"), number="上升下降沿/s") -> (F-format string=w355:string)  [unwired: 2 in]
            n163 = Concatenate Strings(w356, w362, w354, w355) -> (w359:string)
            n164 = VISA Write(VISA resource name=w353, write buffer=w359, error in (no error)=w352) -> (VISA resource name out=w351:refnum<visa-resource-name>, error out=w350:errorcluster)  [unwired: 1 out]
          }
        }
        n165 = VISA Close(VISA resource name=w268, error in (no error)=w267) -> (error out=→"configure error out":errorcluster)
      }
    }
    n166 = event shown="[1] \"Output 1\": 值改变" {
      selector: _ -> [_ _]
      dyn-events: _ -> [_ _]
      timeout: u32 0 ("Time") -> [_ _]
      tunnel: "Output 1" -> [_ w140]
      event Timeout {
        n167 = event-data() -> ()  [unwired: 1 in, 2 out]
      }
      event "Output 1": Value Change {
        n168 = event-data() -> ()  [unwired: 1 in, 6 out]
        n169 = local read "VISA 信号发生器"() -> (w136:refnum<visa-resource-name>)
        n170 = VISA Open(VISA resource name=w136) -> (VISA resource name=w139:refnum<visa-resource-name>, error out=w142:errorcluster)  [unwired: 4 in]
        n171 = stacked-sequence {
          tunnel: w140 -> [w147 _]
          tunnel: w142 -> [w146 _]
          tunnel: w139 -> [w145 _]
          tunnel: [w144 _] -> w138
          tunnel: [w143 _] -> w137
          frame #0 {
            n172 = case shown="真" w147 {
              tunnel: w145 -> [w155 w163]
              tunnel: [w154 w162] -> w143
              tunnel: w146 -> [w153 w160]
              tunnel: [w152 w161] -> w144
              frame True {
                n173 = local write "Output"(TRUE ("布尔")) -> ()
                n174 = local read "channel输出口"() -> (w149:i32)
                n175 = Pick Line(multi-line string=":OUTP1 ON\n:OUTP2 ON" ("write buffer"), line index=w149) -> (output string=w148:string)  [unwired: 1 in]
                n176 = VISA Write(VISA resource name=w155, write buffer=w148, error in (no error)=w153) -> (VISA resource name out=w152:refnum<visa-resource-name>, error out=w154:errorcluster)  [unwired: 1 out]
              }
              frame False {
                n177 = local read "channel输出口"() -> (w157:i32)
                n178 = Pick Line(multi-line string=":OUTP1 OFF\n:OUTP2 OFF" ("write buffer"), line index=w157) -> (output string=w156:string)  [unwired: 1 in]
                n179 = VISA Write(VISA resource name=w163, write buffer=w156, error in (no error)=w160) -> (VISA resource name out=w161:refnum<visa-resource-name>, error out=w162:errorcluster)  [unwired: 1 out]
                n180 = local write "Output"(FALSE ("布尔")) -> ()
              }
            }
          }
          frame #1 {
            n181 = Wait (ms)(milliseconds to wait=u32 150) -> ()  [unwired: 1 out]
          }
        }
        n182 = VISA Close(VISA resource name=w138, error in (no error)=w137) -> (error out=→"output control error  5":errorcluster)
      }
    }
  }
  n183 = flat-sequence {
    frame #0 {
      "Backlight" <- i32[][] [] ("Backlight")
      "data 2" <- i32[][] [] ("data 2")
    }
    frame #1 {
      w365 = FALSE
      # "删除背景光控件\n初始值设定"
      n184 = local write "cut backlight"(w365) -> ()
      "backlight" <- w365
    }
  }
  n185 = stacked-sequence {
    seq-local: [_ _ _ w386 _ _ _ _] -> [_ _ _ _ w404 w424 w427 w532]
    seq-local: [_ _ _ w385 _ _ _ _] -> [_ _ _ _ w405 w425 w426 w533]
    frame #0 {
      # "initialize all variables"
      n186 = property on="initialize" class="Bool"("Désactivé"=u8 0) -> ()  [unwired: 2 in, 2 out]
      n187 = property on="Acquire" class="Bool"("Visible"=FALSE) -> ()  [unwired: 2 in, 2 out]
      n188 = property on="Setup" class="Bool"("Visible"=FALSE) -> ()  [unwired: 2 in, 2 out]
      n189 = local write "indicator"("" ("indicator")) -> ()
      n190 = local write "initialized ?"(FALSE ("initialized ?")) -> ()
      n191 = local write "Continuous"(FALSE ("Continuous")) -> ()
      n192 = local write "Close"(FALSE ("Close")) -> ()
      n193 = property on="Device Name" class="Ring (严格)"("Désactivé"=u8 0) -> ()  [unwired: 2 in, 2 out]
      n194 = property on="Continuous" class="Bool (严格)"("Visible"=FALSE) -> ()  [unwired: 2 in, 2 out]
      n195 = local write "Commande tab"(T1."Settings" ("Commande tab")) -> ()
    }
    frame #1 {
      # "Read Uniq ID"
      n196 = stacked-sequence {
        frame #0 {
          n197 = call <userlib>:"read detector uniq-id.vi"() -> ("nbr of components"=w378:i32, "UniqueID"=w377:string[], "Name"=w376:string[])  [unwired: 4 out]
          n198 = for {
            N: w378 -> [_]
            tunnel: w377 -> [w380]
            tunnel: w376 -> [w379]
            n199 = property on="Device Name" class="Ring (严格)"("Chaînes []"=w379) -> ()  [unwired: 2 in, 2 out]
            n200 = property on="Uniques ID" class="Ring (严格)"("Chaînes []"=w380) -> ()  [unwired: 2 in, 2 out]
          }
        }
      }
    }
    frame #2 {
      n201 = while {
        stop <- "initialize" stop-if-true
        n202 = local read "Device Name"() -> (w383:u16)
        n203 = local write "Uniques ID"(w383) -> ()
        n204 = local read "Close"() -> (w381:bool)
        n205 = Stop(stop? (T)=w381) -> ()
        n206 = Wait Until Next ms Multiple(millisecond multiple=u32 100 ("n millisecondes")) -> ()  [unwired: 1 out]
      }
    }
    frame #3 {
      n207 = stacked-sequence {
        tunnel: [_ w393 _ _] -> w386
        tunnel: [_ w392 _ _] -> w385
        frame #0 {
          n208 = local write "indicator"("Initializing ..." ("indicator")) -> ()
        }
        frame #1 {
          n209 = local read "Uniques ID"() -> (w390:u16)
          n210 = property on="Uniques ID" class="Ring (严格)"() -> ("Chaînes []"=w391:string[])  [unwired: 2 in, 2 out]
          n211 = Index Array(array=w391, index=w390) -> (element=w389:string)
          n212 = call <userlib>:"Initialize CCD.vi"("Unique id:"=w389) -> ("activeYPixels"=→"Y Pixels:":i32, "JYCCDLib.IJYCCDReqd"=w392:refnum<k7>, "activeXPixels"=→"X Pixels:":i32, "sortie d'erreur"=w393:errorcluster, "FirmwareVersion"=→"Firmware\nVersion":string)  [unwired: 3 out]
        }
        frame #2 {
          n213 = property on="initialize" class="Bool"("Désactivé"=u8 2) -> ()  [unwired: 2 in, 2 out]
          n214 = property on="Device Name" class="Ring (严格)"("Désactivé"=u8 2) -> ()  [unwired: 2 in, 2 out]
          n215 = local write "Continuous"(FALSE ("Continuous")) -> ()
          n216 = property on="Setup" class="Bool"("Visible"=TRUE) -> ()  [unwired: 2 in, 2 out]
        }
        frame #3 {
          n217 = local write "initialized ?"(TRUE ("initialized ?")) -> ()
          n218 = local write "indicator"("Initialized !" ("indicator")) -> ()
        }
      }
    }
    frame #4 {
      # "Actually not working"
      # "Read ADC and GAIN"
      n219 = case shown="真" "Constante de condition\n(Voir l'aide contextuelle)" {
        tunnel: w405 -> [_ w415]
        tunnel: w404 -> [_ w414]
        frame False {
        }
        frame True {
          # "Read Input supported trigger"
          n220 = call <userlib>:"Trigger - Get Supported Input.vi"("JYCCDLib.IJYCCDReqd"=w415, "Error Input"=w414) -> ("trigAddress"=w409:i32, "eventPtr"=w410:i32, "trigEventString"=w413:string, "trigSigType"=w412:i32, "trigSigTypeString"=w411:string)  [unwired: 4 out]
          n221 = local write "trigSigTypeString"(w411) -> ()
          n222 = local write "trigAddress"(w409) -> ()
          n223 = local write "Trigger Type :"(w410) -> ()
          n224 = local write "trigEventString"(w413) -> ()
          n225 = local write "Signal type :"(w412) -> ()
        }
      }
      n226 = call <userlib>:"Init ADC & Gain.vi"("JYCCDLib.IJYCCDReqd"=w405, "input error"=w404) -> ("ADC Number"=w403:i32[], "ADC description"=w408:string[], "Gain Number"=w406:i32[], "Gain description"=w407:string[])
      n227 = local write "Gain Number"(w406) -> ()
      n228 = local write "ADC Number"(w403) -> ()
      n229 = stacked-sequence {
        tunnel: w408 -> [w416 _]
        tunnel: w407 -> [_ w417]
        frame #0 {
          n230 = property on="ADC" class="Ring (严格)"("Chaînes []"=w416) -> ()  [unwired: 2 in, 2 out]
        }
        frame #1 {
          n231 = property on="GAIN" class="Ring (严格)"("Chaînes []"=w417) -> ()  [unwired: 2 in, 2 out]
        }
      }
    }
    frame #5 {
      # "IS multi Accumulation Supported ?"
      n232 = call <userlib>:"MultiAccu - Is Supported.vi"("Error In"=w424, "JYCCDLib.IJYCCDReqd"=w425) -> ("IsOperatingModeSupported"=w418:bool)  [unwired: 3 out]
      n233 = Select(t=0, s=w418, f=2) -> (s? t:f=w421:i32)
      n234 = Select(t=FALSE, s=w418, f=w418) -> (s? t:f=w420:bool)
      n235 = local write "Multi Accumulation mode:"(w420) -> ()
      n236 = property on="Multi Accumulation mode:" class="Bool (严格)"("Désactivé"=w421) -> ()  [unwired: 2 in, 2 out]
      n237 = property on="Multi Accumulation mode:" class="Bool (严格)"("Désactivé"=w421) -> ()  [unwired: 2 in, 2 out]
    }
    frame #6 {
      n238 = while {
        tunnel: w426 -> [w434]
        tunnel: w427 -> [w433]
        stop <- "Close" stop-if-true
        n239 = case shown="真" "Reformat" {
          frame False {
          }
          frame True {
            n240 = local read "Y Pixels:"() -> (w510:i32)
            n241 = local read "X Pixels:"() -> (w512:i32)
            n242 = call <userlib>:"Spectral Reformat CCD area.vi"("Y Pixels:"=w510, "X Pixels:"=w512, "numAreas"="Number of Areas :") -> ("areas :"=→"areas :":i32[][])  [unwired: 3 out]
          }
        }
        n243 = case shown="真" "Setup" {
          tunnel: w433 -> [_ w515]
          tunnel: w434 -> [_ w514]
          frame False {
          }
          frame True {
            n244 = stacked-sequence {
              tunnel: w515 -> [_ w529 _]
              tunnel: w514 -> [_ w517 _]
              frame #0 {
                n245 = local write "indicator"("Setting up the detector" ("indicator")) -> ()
              }
              frame #1 {
                w527 = 1 items=["JYMCD_ACQ_FORMAT_IMAGE", "JYMCD_ACQ_FORMAT_SCAN"] ("Acquisition type")
                n246 = local read "Gain Number"() -> (w522:i32[])
                n247 = local read "GAIN"() -> (w518:u16)
                n248 = local read "ADC Number"() -> (w523:i32[])
                n249 = local read "ADC"() -> (w519:u16)
                n250 = Index Array(array=w522, index=w518) -> (element=w520:i32)
                n251 = Index Array(array=w523, index=w519) -> (element=w521:i32)
                n252 = local read "Number of Areas :"() -> (w525:u16)
                n253 = local read "areas :"() -> (w526:i32[][])
                n254 = call <userlib>:"Setup CCD.vi"("numAreas"=w525, "areas :"=w526, "JYCCDLib.IJYCCDReqd"=w517, "entrée d'erreur (pas d'erreur)"=w529, "Acquisition type"=w527, "Gain"=w520, "Select ADC"=w521, "Integration time(ms)"="Integration time (ms) :") -> ("DataSize"=→"DataSize":i32)  [unwired: 1 out]
                "JYCCDLib.IJYCCDReqd" <- w517
              }
              frame #2 {
                w530 = TRUE ("Visible")
                n255 = property on="Continuous" class="Bool (严格)"("Visible"=w530) -> ()  [unwired: 2 in, 2 out]
                n256 = property on="Acquire" class="Bool"("Visible"=w530) -> ()  [unwired: 2 in, 2 out]
                n257 = local write "indicator"("Ready !" ("indicator")) -> ()
              }
            }
          }
        }
        n258 = local read "Continuous"() -> (w435:bool)
        n259 = local read "Accumulations:"() -> (w430:u16)
        n260 = Or(x="Acquire", y=w435) -> (x .or. y?=w432:bool)
        n261 = case shown="真" w432 {
          tunnel: w434 -> [_ w447]
          tunnel: w433 -> [_ w446]
          tunnel: "Enable InputTriggers :" -> [_ w445]
          tunnel: "Multi Accumulation mode:" -> [_ w444]
          tunnel: w430 -> [_ w443]
          tunnel: "MultiAcqShutterMode" -> [_ w442]
          frame False {
          }
          frame True {
            n262 = stacked-sequence {
              seq-local: [_ _ w460 _ _] -> [_ _ _ w490 _]
              tunnel: w447 -> [_ w449 w464 w489 _]
              tunnel: w446 -> [_ w450 w463 w488 _]
              tunnel: w445 -> [_ w451 _ _ _]
              tunnel: w444 -> [_ _ w462 _ _]
              tunnel: w443 -> [_ _ w461 _ _]
              tunnel: w442 -> [_ _ w459 _ _]
              frame #0 {
                n263 = local write "CCD Busy"(TRUE ("CCD Busy")) -> ()
              }
              frame #1 {
                n264 = case shown="真" w451 {
                  tunnel: w450 -> [w452 w458]
                  tunnel: w449 -> [w453 w457]
                  frame False {
                    n265 = call <userlib>:"Trigger - Disable.vi"("Error In"=w452, "JYCCDLib.IJYCCDReqd"=w453) -> ()  [unwired: 6 out]
                  }
                  frame True {
                    n266 = local read "Trigger Type :"() -> (w454:u16)
                    n267 = local read "Signal type :"() -> (w455:enum16{"TTL Rising Edge", "TTL Falling Edge"})
                    n268 = local read "trigAddress"() -> (w456:i32)
                    n269 = call <userlib>:"Trigger - Enable.vi"("Error In"=w458, "sigType"=w455, "event"=w454, "trigAddress"=w456, "JYCCDLib.IJYCCDReqd"=w457) -> ()  [unwired: 3 out]
                  }
                }
              }
              frame #2 {
                n270 = case shown="真" w462 {
                  selector: w462 -> [_ w470]
                  tunnel: w464 -> [w467 w473]
                  tunnel: w463 -> [w466 w472]
                  tunnel: w461 -> [_ w471]
                  tunnel: [u16 1 ("Accumulations:") w471] -> w460
                  tunnel: w459 -> [_ w469]
                  frame False {
                    n271 = call <userlib>:"MultiAccu - Disable.vi"("Error In"=w466, "JYCCDLib.IJYCCDReqd"=w467) -> ()  [unwired: 4 out]
                  }
                  frame True {
                    n272 = call <userlib>:"MultiAccu - Configure.vi"("JYCCDLib.IJYCCDReqd"=w473, "Cleans Before"="Number of Cleans", "Accumulations:"=w471, "MultiAcqHardwareMode"=w470, "MultiAcqShutterMode"=w469, "Error In"=w472) -> ()  [unwired: 1 in, 9 out]
                  }
                }
              }
              frame #3 {
                n273 = local read "cut backlight"() -> (w475:bool)
                n274 = local read "backlight"() -> (w474:bool)
                n275 = call <userlib>:"MultiAccu - Acquire spectral.vi"("error in"=w488, "Accumulations:"=w490, "ShutterOpen"="ShutterOpen", "JYCCDLib.IJYCCDReqd"=w489) -> ("Acq Time(ms)"=→"Acq Time(ms)":u32, "Array Out"=w487:i32[][][])  [unwired: 1 out]
                n276 = And(x=w475, y=w474) -> (x .and. y?=w476:bool)
                n277 = call <userlib>:"Array reset dimension.vi"("Area Number"="Area Number to Display", "Array In"=w487) -> ("Array Out"=w477:i32[][])
                n278 = case shown="真" w476 {
                  tunnel: [w493 w494] -> w478
                  tunnel: w477 -> [w493 w495]
                  frame False {
                  }
                  frame True {
                    n279 = local read "Backlight"() -> (w496:i32[][])
                    n280 = Subtract(x=w495, y=w496) -> (x-y=w494:i32[][])
                  }
                }
                n281 = local write "Data"(w477) -> ()
                n282 = local write "data 2"(w477) -> ()
                n283 = local read "波长范围"() -> (w481:dbl[])
                n284 = Index Array(array=w478, index (row)=0 ("禁用的索引 (列)")) -> (element=w480:i32[])  [unwired: 1 in]
                n285 = Reverse 1D Array(array=w480) -> (reversed array=w479:i32[])
                n286 = call "转换至动态数据2"("Array"=w481) -> ("Dynamic Data Type"=w483:dynamicdata)  [unwired: 3 in]
                n287 = call "转换至动态数据"("Array"=w479) -> ("Dynamic Data Type"=w484:dynamicdata)  [unwired: 3 in]
                n288 = call "Build XY Graph2"("Y Input"=w484, "X Input"=w483) -> ("XY Graph"=w482:cluster{"Y":dbl[], "Y":dbl[]}[])  [unwired: 8 in, 1 out]
                n289 = local write "Spectrum"(w482) -> ()
              }
              frame #4 {
                n290 = case shown="真" "Save Backlight" {
                  frame False {
                  }
                  frame True {
                    w499 = TRUE ("删除背景光")
                    n291 = local read "Data"() -> (w501:i32[][])
                    n292 = local write "Backlight"(w501) -> ()
                    n293 = local write "cut backlight"(w499) -> ()
                    n294 = local write "backlight"(w499) -> ()
                    n295 = local write "Save Backlight"(FALSE ("Save Backlight")) -> ()
                  }
                }
                n296 = local write "CCD Busy"(FALSE ("CCD Busy")) -> ()
              }
            }
          }
        }
        n297 = case shown="真" "Temperature" {
          tunnel: w434 -> [_ w504]
          tunnel: w433 -> [_ w503]
          frame False {
            n298 = property on="temp graph" class="WFChart (严格)"("Visible"=FALSE) -> ()  [unwired: 2 in, 2 out]
          }
          frame True {
            n299 = stacked-sequence {
              tunnel: w504 -> [_ w509]
              tunnel: w503 -> [_ w508]
              frame #0 {
                n300 = property on="temp graph" class="WFChart (严格)"("Visible"=TRUE) -> ()  [unwired: 2 in, 2 out]
              }
              frame #1 {
                w507 = u16 0 items=["° Celsius", "Kelvin", "° Farenheit"] ("units")
                n301 = call <userlib>:"read temperature.vi"("entrée d'erreur (pas d'erreur)"=w508, "units"=w507, "JYCCDLib.IJYCCDReqd"=w509) -> ("Current Temperature"=w506:dbl)
                n302 = local write "temp graph"(w506) -> ()
              }
            }
          }
        }
        n303 = Wait Until Next ms Multiple(millisecond multiple=u32 50 ("n millisecondes")) -> ()  [unwired: 1 out]
      }
    }
    frame #7 {
      n304 = Close Reference(reference=w533, error in (no error)=w532) -> ()  [unwired: 1 out]
    }
  }
  n305 = stacked-sequence {
    seq-local: [_ _ w543 _ _] -> [_ _ _ w553 w558]
    seq-local: [_ _ w542 _ _] -> [_ _ _ w552 _]
    seq-local: [_ _ _ w551 _] -> [_ _ _ _ _]
    frame #0 {
      n306 = call <userlib>:"Get Monos From Config Browser.vi"() -> ("UniqueIDs"=w538:string[], "Mono ID"=w539:string[])  [unwired: 3 in, 1 out]
      n307 = Build Cluster Array(w539, w538) -> (w536:cluster{"String":string, "String":string}[])
      n308 = property on="Mono ID" class="CmbBox"("Strings And Values []"=w536) -> ()  [unwired: 2 in, 2 out]
      n309 = Index Array(array=w536, index=0) -> (element=w537:cluster{"String":string, "String":string})
      n310 = Unbundle(w537) -> ("String"=w534:string)  [unwired: 1 out]
      "Current UniqueID" <- w534
      n311 = local write "Mono ID"(w534) -> ()
    }
    frame #1 {
      n312 = while {
        stop <- "Connect" stop-if-true
        n313 = local read "Mono ID"() -> (w540:string)
        n314 = local write "Current UniqueID"(w540) -> ()
      }
    }
    frame #2 {
      n315 = local read "Mono ID"() -> (w545:string)
      n316 = call <userlib>:"JYInitMono.vi"("Unique ID"=w545, "Force Init"="Force\nInitialization") -> ("Refnum out"=w543:refnum<k7>, "Initialized"=→"Initialized JY":bool, "error out"=w542:errorcluster)  [unwired: 9 in, 2 out]
    }
    frame #3 {
      n317 = call <userlib>:"Show Current Grating.vi"("Refnum in"=w553, "error in (no error)"=w552) -> ("Gratings"=w554:dbl[], "Grating Index"=w548:i32, "Current Grating"=w550:dbl, "Current Description"=w547:string, "error out"=w551:errorcluster)  [unwired: 5 in, 4 out]
      "Gratings" <- w554
      n318 = local write "Current Grating"(w550) -> ()
      n319 = local write "Current Description"(w547) -> ()
      n320 = Number To Decimal String(number=w554) -> (decimal integer string=w556:string[])  [unwired: 1 in]
      n321 = Number To Decimal String(number=w548) -> (decimal integer string=w549:string)  [unwired: 1 in]
      n322 = property on="Target Grating" class="CmbBox"("Value"=w549) -> ()  [unwired: 2 in, 2 out]
      n323 = Build Cluster Array(w556, string[] ["1", "2", "3"]) -> (w557:cluster{"Numeric":string, string}[])
      n324 = property on="Target Grating" class="CmbBox"("Strings And Values []"=w557) -> ()  [unwired: 2 in, 2 out]
    }
    frame #4 {
      n325 = while {
        tunnel: w558 -> [w560]
        stop <- w559 stop-if-true
        n326 = stacked-sequence {
          seq-local: [w564 _ _ _ _] -> [_ w571 w582 _ w589]
          seq-local: [w563 _ _ _ _] -> [_ w570 w581 _ _]
          seq-local: [_ w569 _ _ _] -> [_ _ _ _ _]
          seq-local: [_ w568 _ _ _] -> [_ _ _ _ _]
          seq-local: [_ _ w574 _ _] -> [_ _ _ _ _]
          seq-local: [_ _ w573 _ _] -> [_ _ _ w584 _]
          tunnel: w560 -> [w562 _ _ w585 _]
          frame #0 {
            n327 = call <userlib>:"Show Current Grating.vi"("Refnum in"=w562) -> ("Grating Index"=→"Grating Index":i32, "Current Grating"=→"Current Grating":dbl, "Current Description"=→"Current Description":string, "error out"=w563:errorcluster, "JYMONOLib.IJYMonoReqd"=w564:refnum<k7>)  [unwired: 6 in, 4 out]
          }
          frame #1 {
            n328 = call <userlib>:"JYGetCurrentWL.vi"("error in (no error)"=w570, "JYMONOLib.IJYMonoReqd"=w571) -> ("error out"=w568:errorcluster, "Units"=→"Units":string, "Current WL"=→"Current WL":dbl, "JYMONOLib.IJYMonoReqd 2"=w569:refnum<k7>)  [unwired: 6 in]
          }
          frame #2 {
            w579 = u16 1 items=["Entrance", "Exit"] ("Mirror Number")
            w580 = u16 0 items=["Entrance", "Exit"] ("Mirror Number")
            n329 = call <userlib>:"JYGetMirrorPos.vi"("error in (no error)"=w581, "Mirror"=w580, "Refnum In"=w582) -> ("error out"=w577:errorcluster, "Current Mirror Position"=→"Entrance Mirror\nPosition":i32, "Refnum Out"=w578:refnum<k7>)  [unwired: 1 in]
            n330 = call <userlib>:"JYGetMirrorPos.vi"("error in (no error)"=w577, "Mirror"=w579, "Refnum In"=w578) -> ("error out"=w573:errorcluster, "Current Mirror Position"=→"Exit Mirror\nPosition":i32, "Refnum Out"=w574:refnum<k7>)  [unwired: 1 in]
          }
          frame #3 {
            w587 = u16 0 items=["Front Entrance", "Side Entrance", "Front Exit", "Side Exit", "First Intermediate", "Second Intermediate"] ("Slit")
            n331 = call <userlib>:"JYGetSlits.vi"("MonoRefNum IN"=w585, "Slit"=w587, "error in (no error)"=w584) -> ("Units"=→"Units 2":string, "Slit Width"=→"Front Entrance":dbl, "error out"=→"error out":errorcluster)  [unwired: 13 in, 1 out]
          }
          frame #4 {
            n332 = local read "Move To\nTarget Positions"() -> (w590:bool)
            n333 = case shown="真" w590 {
              tunnel: w589 -> [_ w591]
              frame False {
              }
              frame True {
                n334 = stacked-sequence {
                  seq-local: [w593 _ _ _] -> [_ w599 _ _]
                  seq-local: [_ w597 _ _] -> [_ _ w614 _]
                  seq-local: [_ _ w601 _] -> [_ _ _ w620]
                  seq-local: [_ _ _ w617] -> [_ _ _ _]
                  tunnel: w591 -> [w595 w598 w612 w621]
                  frame #0 {
                    n335 = property on="Target Grating" class="CmbBox"() -> ("Value"=w592:string)  [unwired: 2 in, 2 out]
                    n336 = local read "error out"() -> (w594:errorcluster)
                    n337 = Decimal String To Number(string=w592) -> (number=w596:i32)  [unwired: 2 in, 1 out]
                    n338 = call <userlib>:"JYTurret.vi"("error in (no error)"=w594, "Grating Index"=w596, "JYMONOLib.IJYMonoReqd"=w595) -> ("error out"=w593:errorcluster)  [unwired: 2 out]
                  }
                  frame #1 {
                    # "Move Grating to Target Position"
                    n339 = call <userlib>:"JYMoveToWavelength.vi"("error in (no error)"=w599, "Target WL"="Target WL", "RefNum In"=w598) -> ("error out"=w597:errorcluster)  [unwired: 1 in, 2 out]
                  }
                  frame #2 {
                    w607 = u16 1 items=["Entrance", "Exit"] ("Mirror Number")
                    w606 = u16 0 items=["Entrance", "Exit"] ("Mirror Number")
                    w613 = u16 1 items=["Entrance", "Exit", "Front", "Side"] ("Mirror Number")
                    w616 = u16 0 items=["Entrance", "Exit", "Front", "Side"] ("Mirror Number")
                    # "Move Mirrors"
                    n340 = call <userlib>:"JYMirrorMove.vi"("error in (no error)"=w614, "Mirror Position"="Entrance Mirror", "Mirror Number"=w616, "RefNum In"=w612) -> ("error out"=w611:errorcluster)  [unwired: 6 in, 1 out]
                    n341 = call <userlib>:"JYMirrorMove.vi"("error in (no error)"=w611, "Mirror Position"="Exit Mirror", "Mirror Number"=w613, "RefNum In"=w612) -> ("error out"=w604:errorcluster, "MonoRefNum Out"=w605:refnum<k7>)  [unwired: 6 in]
                    n342 = call <userlib>:"JYGetMirrorPos.vi"("error in (no error)"=w604, "Mirror"=w606, "Refnum In"=w605) -> ("error out"=w609:errorcluster, "Current Mirror Position"=w603:i32, "Refnum Out"=w608:refnum<k7>)  [unwired: 1 in]
                    n343 = local write "Entrance Mirror\nPosition"(w603) -> ()
                    n344 = call <userlib>:"JYGetMirrorPos.vi"("error in (no error)"=w609, "Mirror"=w607, "Refnum In"=w608) -> ("error out"=w601:errorcluster, "Current Mirror Position"=w602:i32)  [unwired: 1 in, 1 out]
                    n345 = local write "Exit Mirror\nPosition"(w602) -> ()
                  }
                  frame #3 {
                    w619 = u16 0 items=["Front Entrance", "Side Entrance", "Front Exit", "Side Exit", "First Intermediate", "Second Intermediate"] ("Slit")
                    # "Set New Slit Positions"
                    n346 = call <userlib>:"JYSlits.vi"("JYMONOLib.IJYMonoReqd"=w621, "Slit"=w619, "error in (no error)"=w620, "Slit Width"="Target\nFront Entrance") -> ("error out"=w617:errorcluster)  [unwired: 1 in, 1 out]
                  }
                }
              }
            }
          }
        }
        n347 = local read "Close"() -> (w559:bool)
      }
    }
  }
  n348 = for {
    N: 1024 -> [_]
    tunnel: [w626] -> w3 mode=indexing
    i -> [w628]
    n349 = Subtract(x="终止波长", y="起始波长") -> (x-y=w624:dbl)
    n350 = Divide(x=w624, y=1024.0) -> (x/y=w622:dbl)
    n351 = Multiply(x=w622, y=w628) -> (x*y=w627:dbl)
    n352 = Add(x=w627, y="起始波长") -> (x+y=w626:dbl)
  }
  "波长范围" <- w3
